vi "sub_DTMF_Dequantize_BitDecoding.vi"(8 "bitLength":i32, 9 "GrayCode":bool, 10 "L":u16=16 min=2, 11 "RXbitStream":i32[](array[numeric])) -> (3 "dequants":dbl[](array[numeric]))   [LabVIEW 2011]
uses:
  <vilib>/imath/engines/lvmath2/RunTimeEngine/ErrorHandling/NIMS_Finalize Error.vi
  <vilib>/imath/engines/lvmath2/RunTimeEngine/BuiltInFunctions/log2/NIMS_log2(1o).vi
  <instcachedir>/0/NIMS_log2(1o)_7A1FF839A5EC4375BBB20124C6B1C03A.lvgen/NIMS_log2(1o)_7A1FF839A5EC4375BBB20124C6B1C03A_001.vi
  <vilib>/imath/engines/lvmath2/RunTimeSupport/NIMS_Complex To Real.vi
  <instcachedir>/0/NIMS_Complex To Real_C6C689ECDA084B0290AC275552CC3682.lvgen/NIMS_Complex To Real_C6C689ECDA084B0290AC275552CC3682_001.vi
  <vilib>/imath/engines/lvmath2/RunTimeEngine/BuiltInFunctions/reshapemx/NIMS_[GM]_reshapemx.vi
  <instcachedir>/0/NIMS_[GM]_reshapemx_12D4325B6A364072A466707E3686FAB8.lvgen/NIMS_[GM]_reshapemx_12D4325B6A364072A466707E3686FAB8_005.vi
  <vilib>/imath/engines/lvmath2/RunTimeEngine/ErrorHandling/NIMS_Create Error From Enums.vi
  <vilib>/imath/engines/lvmath2/RunTimeEngine/NodeEndStatement/NIMS_NodeEndStatement_Get Vector.vi
  <instcachedir>/0/NIMS_NodeEndStatement_Get Vector_50E2F48DC826428EA11CD85545CBACBE.lvgen/NIMS_NodeEndStatement_Get Vector_50E2F48DC826428EA11CD85545CBACBE_001.vi
  <vilib>/imath/engines/lvmath2/RunTimeEngine/NodeEndStatement/NIMS_NodeEndStatement_Output.vi
  <instcachedir>/0/NIMS_NodeEndStatement_Output_53EC0D466D134D7ABD903AC30B43404B.lvgen/NIMS_NodeEndStatement_Output_53EC0D466D134D7ABD903AC30B43404B_005.vi
  <vilib>/imath/engines/lvmath2/RunTimeEngine/RangeToken/NIMS_Range.vi
  <instcachedir>/0/NIMS_Range_0B7635FB69F84E19AA68E7FF959DF37C.lvgen/NIMS_Range_0B7635FB69F84E19AA68E7FF959DF37C_001.vi
  <vilib>/imath/engines/lvmath2/RunTimeEngine/ArithmeticOperatorToken/NIMS_ArithmeticOperator_multmx(RV,M).vi
  <instcachedir>/0/NIMS_ArithmeticOperator_multmx(RV,M)_0F69384DF375434AAFCFC7849B80E797.lvgen/NIMS_ArithmeticOperator_multmx(RV,M)_0F69384DF375434AAFCFC7849B80E797_001.vi
  <vilib>/imath/engines/lvmath2/RunTimeEngine/VariableToken/Read/NIMS_Get Elements - RV(_) - Check(_).vi
  <instcachedir>/0/NIMS_Get Elements - RV(_) - Check(_)_95E78A4FFA0646428F3543E57837F638.lvgen/NIMS_Get Elements - RV(_) - Check(_)_95E78A4FFA0646428F3543E57837F638_000.vi
  <vilib>/imathl/engines/lvmath/Functions/Error Handling/Create Error.vi
  <vilib>/imath/engines/lvmath2/RunTimeEngine/VariableToken/NIMS_VariableToken_CondDefined.vi
  <instcachedir>/0/NIMS_VariableToken_CondDefined_D30D2F4D3CE04567BC79CC35D27951F7.lvgen/NIMS_VariableToken_CondDefined_D30D2F4D3CE04567BC79CC35D27951F7_001.vi
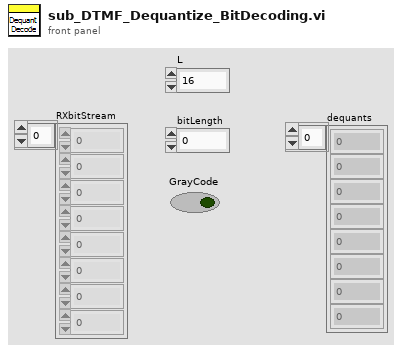
[diagram p1: front panel]
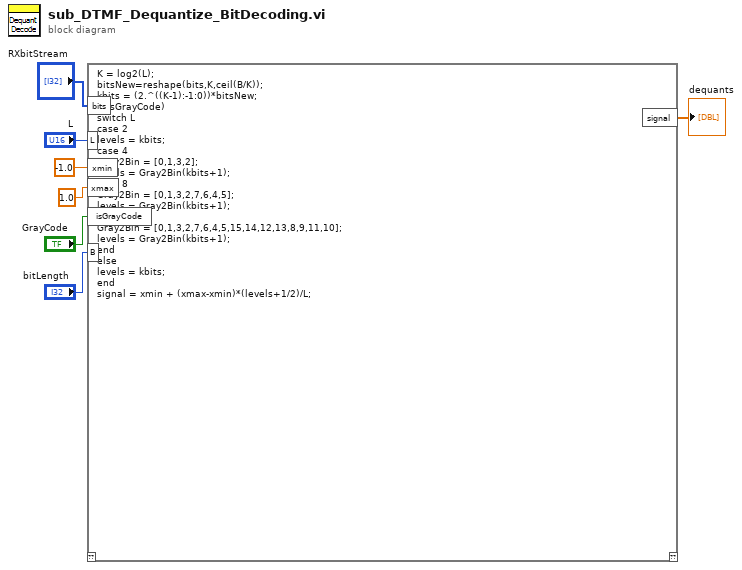
[diagram p0: block diagram]
diagram:
  n1 = mathscript code="K = log2(L);\nbitsNew=reshape(bits,K,ceil(B/K));\nkbits = (2.^((K-1):-1:0))*bitsNew;\nif(isGrayCode)\nswitch L\ncase 2\nlevels = kbits;\ncase 4\nGray2Bin = [0,1,3,2];\nlevels = Gray2Bin(kbits+1);\ncase 8\nGray2Bin = [0,1,3,2,7,6,4,5];\nlevels = Gray2Bin(kbits+1);\ncase 16\nGray2Bin = [0,1,3,2,7,6,4,5,15,14,12,13,8,9,11,10];\nlevels = Gray2Bin(kbits+1);\nend\nelse\nlevels = kbits;\nend\nsignal = xmin + (xmax-xmin)*(levels+1/2)/L;"("L"="L", "isGrayCode"="GrayCode", "bits"="RXbitStream", "B"="bitLength", "xmin"=-1.0, "xmax"=1.0) -> ("signal"=→"dequants":dbl[])  [unwired: 1 in, 1 out]
